vi "Test Handle Command.vi"() -> ()   [LabVIEW 2019, in "Instrument.Lockin.lvlib" / "Instrument.Lockin.lvclass"]
uses:
  Instrument.Lockin.lvclass
  Typedefs/API/Lockin.Commands--Enum.ctl
  Typedefs/API/Lockin.Commands.Local--Enum.ctl
  2f52ef36-3366-4c54-815e-7add623a24a6.vi
  <vilib>/Utility/Data Type/Get Type Information.vi
  <vilib>/Utility/Data Type/Get Numeric Information.vi
  <userlib>/_OpenG.lib/lvdata/lvdata.llb/Unwrap VVariant__ogtk.vi
panel:
  out "Array":T1(array[cluster])
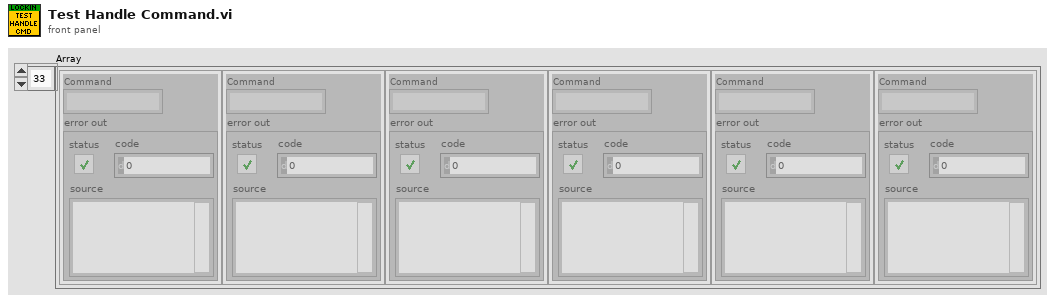
[diagram p1: front panel]
types:
  T1 = cluster{"Command":string, "error out":errorcluster}[]
  T2 = typedef "Instrument.Lockin.lvlib/Instrument.Lockin.lvclass/Lockin.Commands.Local--Enum.ctl" = enum16{"autoConfigureDAQ", "setSimulationMode", "zeroPhase", "setCalibration", "setPreFilter", "setLinkFrequencies", "setLimitAmplitude", "setSamplingDecimationPreDSP", "setSamplingDecimationPostDSP", "setSamplingMode", "setSamplingFsMultiplier", "setSamplingFsOutput", "setSamplingRefreshRate", "setData_State", "setData_DAQ", "setData_Sampling", "setData_Waveforms", "setData_Results", "setData_SweepWaveforms", "setData_AIChannels", "setData_AOChannels", "setData_REFChannels", "setData_InputGain", "setData_OutputGain", "showUI", "setAI", "setOffset", "setOffsetMode"}
  T3 = typedef "Instrument.Lockin.lvlib/Instrument.Lockin.lvclass/Lockin.Commands--Enum.ctl" = enum16{"setAO", "setAO_Amplitude", "setAO_DC", "setAO_Frequency", "setAO_Phase", "setAO_Function", "setREF", "setREF_Frequency", "setREF_Phase", "setREF_TC", "setREF_Roll-Off", "setDAQ", "setSampling", "setState", "getState", "getAO", "getAI", "getResults", "getSampling", "getAOconfig", "getREFconfig", "setInputGain", "setOutputGain", "getInputGain", "getOutputGain", "setSamplingFsMode", "getSamplingFsMode", "setSweep", "setSweep_Time", "setSweep_Table", "getStatus", "getSweepResults", "getSweepWaveforms", "startLogging", "stopLogging"}
  T4 = cluster{"Command":string, "error out":errorcluster}
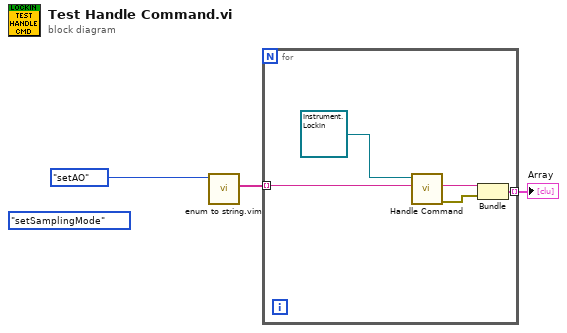
[diagram p0: block diagram]
diagram:
  (unwired) Lockin.Commands.Local--Enum."setSamplingMode" ("Enum")
  n1 = call "enum to string.vim"("enum in"=Lockin.Commands--Enum."setAO" ("Commands")) -> ("strings out"=w3:string[])  [unwired: 9 in, 1 out]
  n2 = for {
    tunnel: w3 -> [w7] mode=indexing
    tunnel: [w4] -> w2 mode=indexing
    n3 = call-dynamic "Handle Command.vi"("Command"=w7, "Instrument.Lockin"=refnum<class "Instrument.Lockin.lvclass"> refnum) -> ("error out"=w5:errorcluster, "Command"=w6:string)  [unwired: 6 in, 2 out]
    n4 = Bundle("Command"=w6, "error out"=w5) -> (w4:T4)  [unwired: 1 in]
  }
  "Array" <- w2
